vi "ExtractCtlsInPages.vi"(8 "error in (no error)":errorcluster, 11 "Ctl Array":refnum<vi>[](array[refnum])) -> (0 "error out":errorcluster, 3 "Ctl Extracted Array":refnum<vi>[](array[refnum]))   [LabVIEW 2015]
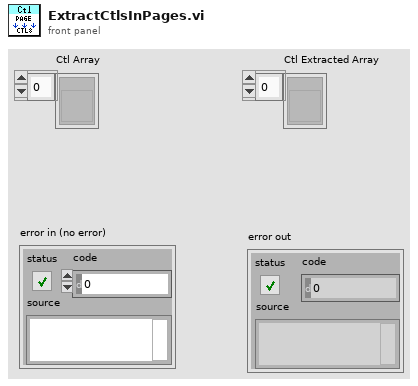
[diagram p1: front panel]
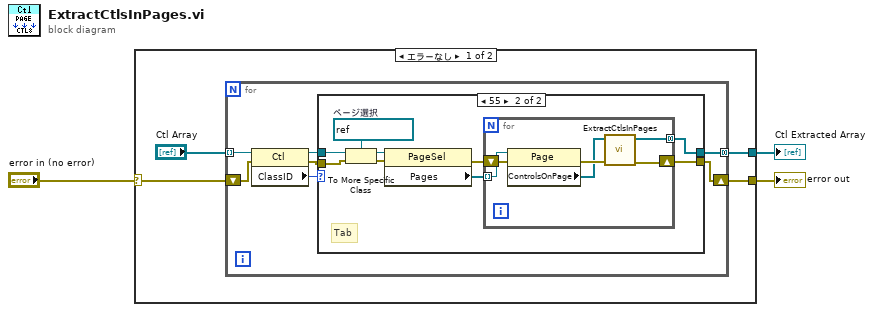
[diagram p0: block diagram]
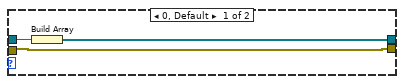
[diagram p2: hidden frame]
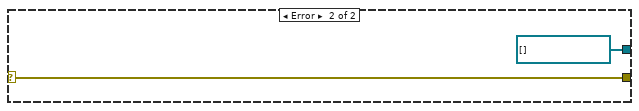
[diagram p3: hidden frame]
diagram:
  n1 = case shown="エラーなし" "error in (no error)" {
    selector: "error in (no error)" -> [w5 w33]
    tunnel: [w6 refnum<vi>[] [] ("Ctl Extracted Array")] -> w2
    tunnel: [w4 w33] -> w1
    frame No Error {
      n2 = for {
        tunnel: "Ctl Array" -> [w14] mode=indexing
        tunnel: [w10] -> w6 mode=concatenating
        shift-right: [w8] -> w4
        shift-left: w5 -> [w9]
        n3 = property class="Ctl"(reference=w14, error in=w9) -> (reference out=w12:refnum<vi>, error out=w11:errorcluster, "ClassID"=w13:u32)
        n4 = case shown="55" w13 {
          tunnel: w12 -> [w17 w25]
          tunnel: w11 -> [w15 w24]
          tunnel: [w16 w19] -> w10
          tunnel: [w15 w18] -> w8
          frame 0, Default {
            n5 = Build Array(w17) -> (w16:refnum<vi>[])
          }
          frame 55 {
            w26 = refnum<vi> refnum  # ページ選択
            # "Tab"
            n6 = To More Specific Class(target class=w26, reference=w25, error in=w24) -> (specific class reference=w23:refnum<vi>, error out=w22:errorcluster)
            n7 = property class="PageSel"(reference=w23, error in=w22) -> (error out=w20:errorcluster, "Pages"=w21:refnum<vi>[])  [unwired: 1 out]
            n8 = for {
              tunnel: w21 -> [w32] mode=indexing
              shift-right: [w28] -> w18
              shift-left: w20 -> [w31]
              tunnel: [w27] -> w19 mode=concatenating
              n9 = property class="Page"(reference=w32, error in=w31) -> (error out=w30:errorcluster, "ControlsOnPage"=w29:refnum<vi>[])  [unwired: 1 out]
              n10 = call "ExtractCtlsInPages.vi"("error in (no error)"=w30, "Ctl Array"=w29) -> ("error out"=w28:errorcluster, "Ctl Extracted Array"=w27:refnum<vi>[])  [unwired: 8 in]
            }
          }
        }
      }
    }
    frame Error {
    }
  }
  "error out" <- w1
  "Ctl Extracted Array" <- w2
